vi "Setup Master.vi"(8 "error in (no error)":errorcluster, 9 "Measurment Time(s)":dbl, 10 "Pre-Trigger Time(s)":dbl, 11 "Master Counter":tag) -> (0 "error out":errorcluster, 2 "Timebase":string, 3 "Master Task out":refnum<k21>)   [LabVIEW 2015]
uses:
  <vilib>/DAQmx/create/channels.llb/DAQmx Create Channel (CO-Pulse Generation-Time).vi
  <vilib>/DAQmx/configure/trigger.llb/DAQmx Start Trigger (None).vi
  <vilib>/DAQmx/configure/timing.llb/DAQmx Timing (Implicit).vi
  <resource>/objmgr/daqmx.rc
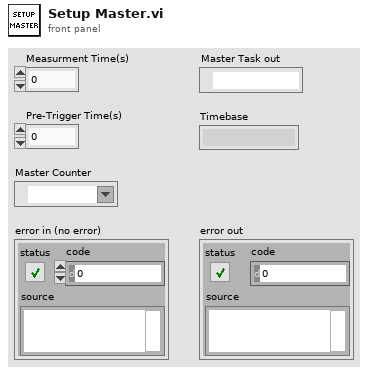
[diagram p1: front panel]
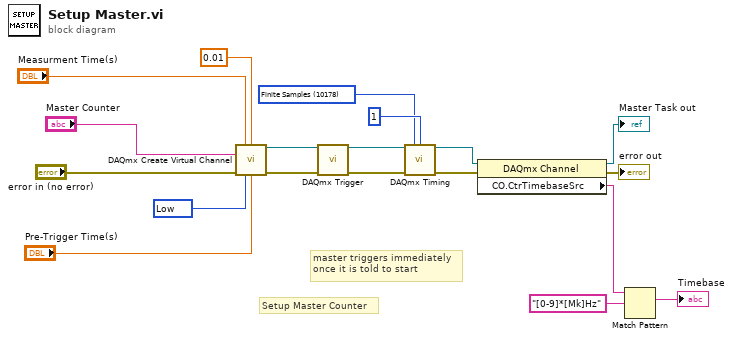
[diagram p0: block diagram]
diagram:
  w4 = 10178 items=["Finite Samples"=10178, "Continuous Samples"=10123, "Hardware Timed Single Point"=12522] ("sample mode")
  w3 = 10214 items=["High"=10192, "Low"=10214] ("idle state")
  # "Setup Master Counter"
  # "master triggers immediately\nonce it is told to start"
  n1 = call-poly <vilib>:"DAQmx Create Virtual Channel.vi"("high time"="Measurment Time(s)", "low time"=0.01, "counter"="Master Counter", "error in"="error in (no error)", "idle state"=w3, "initial delay"="Pre-Trigger Time(s)") -> ("task out"=w6:refnum<k21>, "error out"=w7:errorcluster)  [unwired: 8 in]
  n2 = call-poly <vilib>:"DAQmx Trigger.vi"("task/channels in"=w6, "error in"=w7) -> ("task out"=w8:refnum<k21>, "error out"=w9:errorcluster)  [unwired: 12 in]
  n3 = call-poly <vilib>:"DAQmx Timing.vi"("task/channels in"=w8, "sample mode"=w4, "samples per channel"=1, "error in"=w9) -> ("task out"=w12:refnum<k21>, "error out"=w15:errorcluster)  [unwired: 10 in]
  n4 = property class="DAQmx Channel"(reference=w12, error in=w15) -> (reference out=→"Master Task out":refnum<k21>, error out=→"error out":errorcluster, "CO.CtrTimebaseSrc"=w17:tag)
  n5 = Match Pattern(string=w17, regular expression="[0-9]*[Mk]Hz") -> (match substring=→"Timebase":string)  [unwired: 1 in, 3 out]
